vi "Write Message to Tool.vi"(8 "error in (no error)":errorcluster, 9 "Message Data":variant, 10 "Message":string="Message") -> (0 "error out":errorcluster)   [LabVIEW 2015, in "Tool Interface.lvlib"]
uses:
  Tool Interface.lvlib
  Tool Typedefs/Message Cluster.ctl
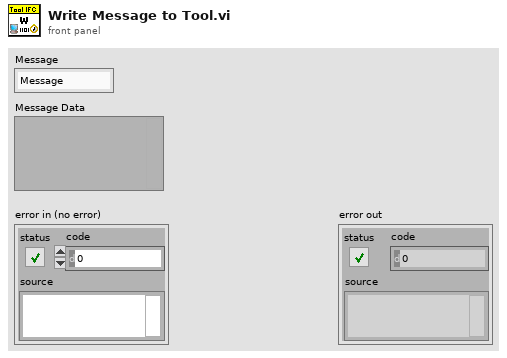
[diagram p1: front panel]
types:
  T1 = typedef "Message Cluster.ctl" = cluster{"Message":string, "Message Data":variant}
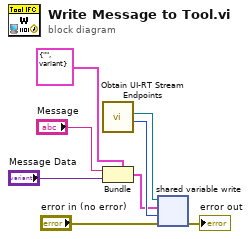
[diagram p0: block diagram]
diagram:
  n1 = call "Obtain UI-RT Stream Endpoints.vi"() -> ("Connect Timeout(ms)"=w8:i32, "UI Command Stream"=w7:refnum<k21>)  [unwired: 9 in, 1 out]
  n2 = Bundle(cluster=T1 {"Message"="", "Message Data"=variant} ("Message Cluster"), "Message"="Message", "Message Data"="Message Data") -> (w6:T1)
  n3 = shared-variable-write(w7, "error in (no error)", w6, w8) -> (→"error out":errorcluster)  [unwired: 2 out]
